vi "Rotation3d_ToRotation2d.vi"(11 "in Rotation3d":T1={"Q_quaternion"={"R"=1.0, "V"=[0.0, 0.0, 0.0]}}) -> (3 "out Rotation2d":T3={"VALUE"=0.0, "COS"=1.0, "SIN"=0.0} {"SIN" format="%13.4f"; "COS" format="%13.4f"; "VALUE" format="%13.4f"})   [LabVIEW 2019, in "Trajectory_Library.lvlib"]
doc: "Returns a Rotation2d representing this Rotation3d projected into the X-Y plane\n\nParameters:\n - IN ROTATION3D -- This ROTATION3D data structure\n\nResults:\n -- out Rotation2d -- A Rotation2d representing this Rotation3d projected into the X-Y plane."
uses:
  Trajectory_Library.lvlib
  TypeDef/QUATERNION.ctl
  TypeDef/ROTATION3D.ctl
  TypeDef/ROTATION2D.ctl
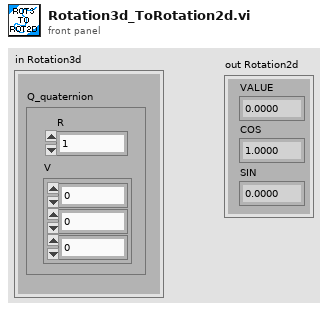
[diagram p1: front panel]
types:
  T1 = typedef "Trajectory_Library.lvlib/ROTATION3D.ctl" = cluster{"Q_quaternion":T2}
  T2 = typedef "Trajectory_Library.lvlib/QUATERNION.ctl" = cluster{"R":dbl, "V":dbl[]}
  T3 = typedef "Trajectory_Library.lvlib/ROTATION2D.ctl" = cluster{"VALUE":dbl, "COS":dbl, "SIN":dbl}
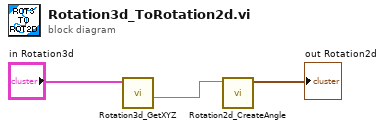
[diagram p0: block diagram]
diagram:
  n1 = call "Rotation3d_GetXYZ.vi"("in Rotation3d"="in Rotation3d") -> ("Z"=w2:dbl)  [unwired: 8 in, 2 out]
  n2 = call "Rotation2d_CreateAngle.vi"("Angle"=w2) -> ("ROTATION"=→"out Rotation2d":T3)  [unwired: 10 in]
